vi "FanGraph.vi"(0 "DeviceControl":refnum<k24>, 1 "Detections":refnum<k24>[](array[refnum])) -> (7 "DeviceControl Out":refnum<k24>)   [LabVIEW 2012]
uses:
  C:/Program Files/LeddarTech/xtec/LeddarNET2.dll
panel:
  out "Angular View":cluster{"Y":dbl[], "Y":dbl[]}[](graph)
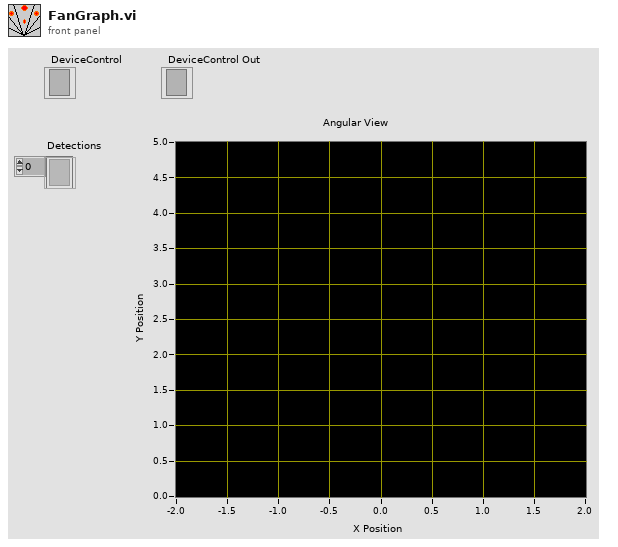
[diagram p1: front panel]
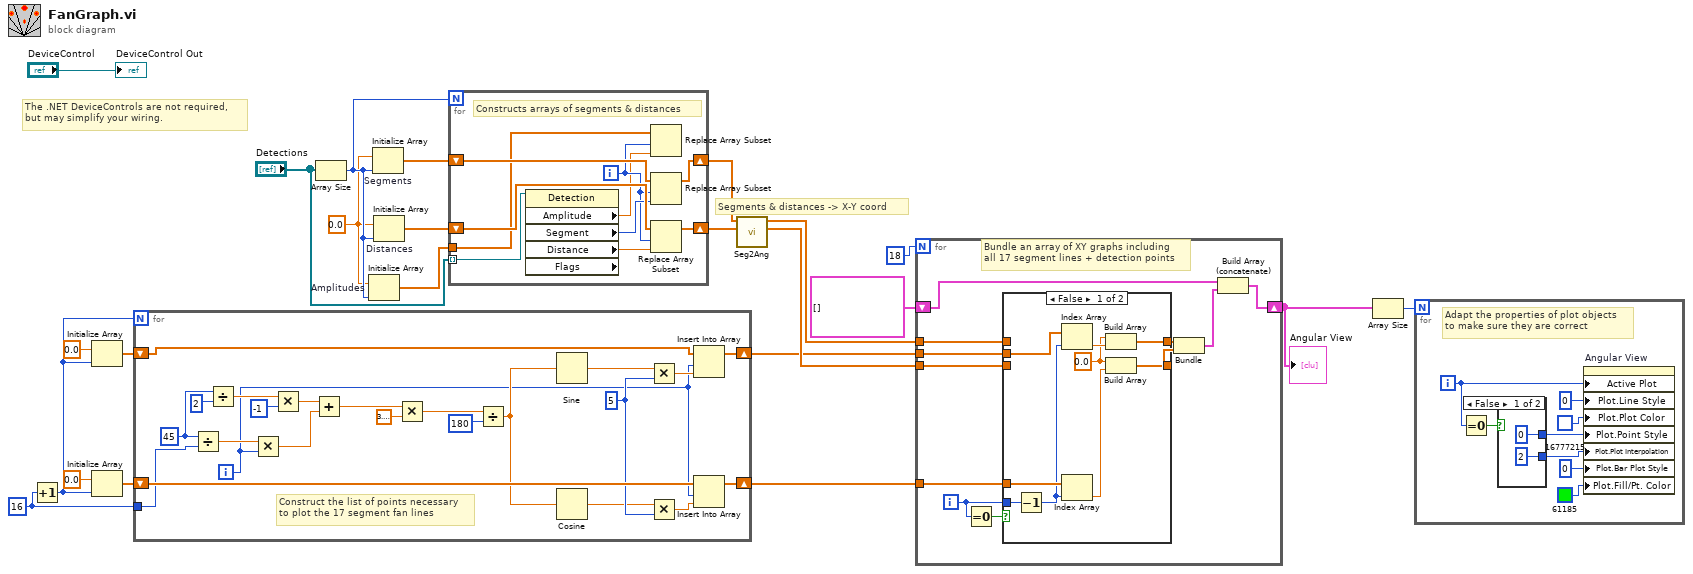
[diagram p0: block diagram]
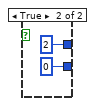
[diagram p2: hidden frame]
diagram:
  w10 = 16 ("dimension size")
  w20 = 0.0 ("element")
  # "The .NET DeviceControls are not required,\nbut may simplify your wiring."
  # "Segments & distances -> X-Y coord"
  n1 = Increment(x=w10) -> (x+1=w11:i32)
  n2 = Initialize Array(0.0 ("element"), w11) -> (w13:dbl[])
  n3 = Initialize Array(0.0 ("element"), w11) -> (w14:dbl[])
  n4 = for {
    N: w11 -> [_]
    shift-right: [w45] -> w6
    shift-left: w14 -> [w46]
    shift-right: [w43] -> w7
    shift-left: w13 -> [w44]
    tunnel: w10 -> [w24]
    i -> [w25]
    w33 = 45
    w36 = 5
    # "Construct the list of points necessary\nto plot the 17 segment fan lines"
    n5 = Divide(x=w33, y=w24) -> (x/y=w32:dbl)
    n6 = Divide(x=w33, y=2 ("dimension size")) -> (x/y=w29:dbl)
    n7 = Multiply(x=w32, y=w25) -> (x*y=w31:dbl)
    n8 = Multiply(x=w29, y=-1 ("dimension size")) -> (x*y=w30:dbl)
    n9 = Add(x=w30, y=w31) -> (x+y=w26:dbl)
    n10 = Multiply(x=w26, y=3.141592653589793) -> (x*y=w41:dbl)
    n11 = Divide(x=w41, y=180) -> (x/y=w40:dbl)
    n12 = Sine(x=w40) -> (sin(x)=w34:dbl)
    n13 = Cosine(x=w40) -> (cos(x)=w35:dbl)
    n14 = Multiply(x=w34, y=w36) -> (x*y=w38:dbl)
    n15 = Multiply(x=w35, y=w36) -> (x*y=w37:dbl)
    n16 = Insert Into Array(array=w44, index=w25, new element=w38) -> (w43:dbl[])
    n17 = Insert Into Array(array=w46, index=w25, new element=w37) -> (w45:dbl[])
  }
  n18 = Array Size(array="Detections") -> (size(s)=w21:i32)
  n19 = Initialize Array "Amplitudes"(w20, w21) -> (w19:dbl[])
  n20 = Initialize Array "Segments"(w20, w21) -> (w22:dbl[])
  n21 = Initialize Array "Distances"(w20, w21) -> (w23:dbl[])
  n22 = for {
    N: w21 -> [_]
    tunnel: "Detections" -> [w56] mode=indexing
    shift-right: [w47] -> w17
    shift-left: w22 -> [w54]
    shift-right: [w48] -> w18
    shift-left: w23 -> [w55]
    tunnel: w19 -> [w50]
    i -> [w51]
    # "Constructs arrays of segments & distances"
    n23 = property class="Detection" props=["Amplitude", "Segment", "Distance", "Flags"](reference=w56) -> ("Amplitude"=w49:sgl, "Segment"=w53:i32, "Distance"=w52:sgl)  [unwired: 1 in, 3 out]
    n24 = Replace Array Subset(array=w50, new element=w49, index=w51) -> ()  [unwired: 1 out]
    n25 = Replace Array Subset(array=w54, new element=w53, index=w51) -> (w47:dbl[])
    n26 = Replace Array Subset(array=w55, new element=w52, index=w51) -> (w48:dbl[])
  }
  n27 = call "Seg2Ang.vi"("Distances"=w18, "Segments"=w17) -> ("Y"=w8:dbl[], "X"=w9:dbl[])  [unwired: 7 in]
  n28 = for {
    N: i16 18 ("y") -> [_]
    tunnel: w9 -> [w66]
    tunnel: w8 -> [w65]
    tunnel: w7 -> [w64]
    tunnel: w6 -> [w63]
    shift-right: [w57] -> w2
    shift-left: cluster{"X":dbl[], "Y":dbl[]}[] [] -> [w58]
    i -> [w62]
    # "Bundle an array of XY graphs including\nall 17 segment lines + detection points"
    n29 = Equal To 0?(x=w62) -> (x = 0?=w67:bool)
    n30 = case shown="False" w67 {
      tunnel: w66 -> [_ w78]
      tunnel: w65 -> [_ w77]
      tunnel: [w72 w78] -> w61
      tunnel: [w70 w77] -> w60
      tunnel: w64 -> [w76 _]
      tunnel: w63 -> [w75 _]
      tunnel: w62 -> [w74 _]
      frame False {
        w68 = 0.0 ("element")
        n31 = Decrement(x=w74) -> (x-1=w73:i32)
        n32 = Index Array "Index Array"(array=w76, index=w73) -> (element=w71:dbl)
        n33 = Index Array(array=w75, index=w73) -> (element=w69:dbl)
        n34 = Build Array "Build Array"(w68, w71) -> (w72:dbl[])
        n35 = Build Array(w68, w69) -> (w70:dbl[])
      }
      frame True {
      }
    }
    n36 = Bundle "Bundle"("X"=w61, "Y"=w60) -> (w59:cluster{"X":dbl[], "Y":dbl[]})  [unwired: 1 in]
    n37 = Build Array (concatenate) "Build Array"(w58, w59) -> (w57:cluster{"X":dbl[], "Y":dbl[]}[])
  }
  "Angular View" <- w2
  n38 = Array Size(array=w2) -> (size(s)=w3:i32)
  n39 = for {
    N: w3 -> [_]
    i -> [w81]
    # "Adapt the properties of plot objects\nto make sure they are correct"
    n40 = Equal To 0?(x=w81) -> (x = 0?=w86:bool)
    n41 = case shown="False" w86 {
      tunnel: [u8 0 ("Plot.Line Style") i16 2 ("y")] -> w85
      tunnel: [i16 2 ("y") i16 0 ("y")] -> w84
      frame False {
      }
      frame True {
      }
    }
    n42 = property on="Angular View" class="XYGraph (strict)"("Active Plot"=w81, "Plot.Line Style"=u8 0, "Plot.Plot Color"=u32 16777215, "Plot.Point Style"=w85, "Plot.Plot Interpolation"=w84, "Plot.Bar Plot Style"=u8 0 ("Plot.Line Style"), "Plot.Fill/Pt. Color"=u32 61185) -> ()  [unwired: 2 in, 2 out]
  }
  "DeviceControl Out" <- "DeviceControl"
